vi "FTW-BuildUtil-PostBuildAction.vi"(5 "Files Generated by Build":path[](array[path]), 6 "Top Level/Always Included VIs":path[](array[path]), 7 "Destination Path":path, 8 "error in (no error)":errorcluster, 9 "Target Name":string, 10 "Build Specification Name":string, 11 "Project Path":path) -> (0 "error out":errorcluster)   [LabVIEW 2013]
uses:
  <userlib>/_OpenG.lib/error/error.llb/Filter Error Codes (Array)__ogtk.vi
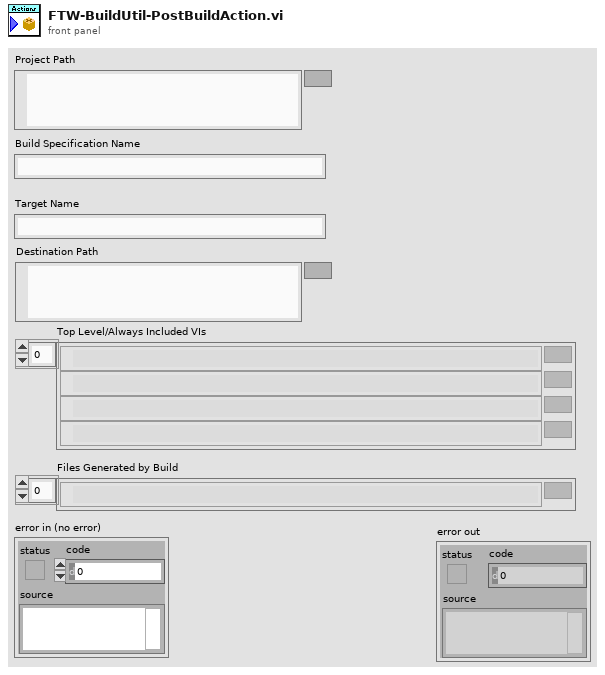
[diagram p1: front panel]
types:
  T1 = cluster{"Major":u16, "Minor":u16, "Fix":u16, "Build":u16}
  T2 = cluster{"Path":path, "lowercase file extension":string, "vi reference":refnum<vi>, "LVClass.Open":refnum<vi>, "Open Library":refnum<vi>}
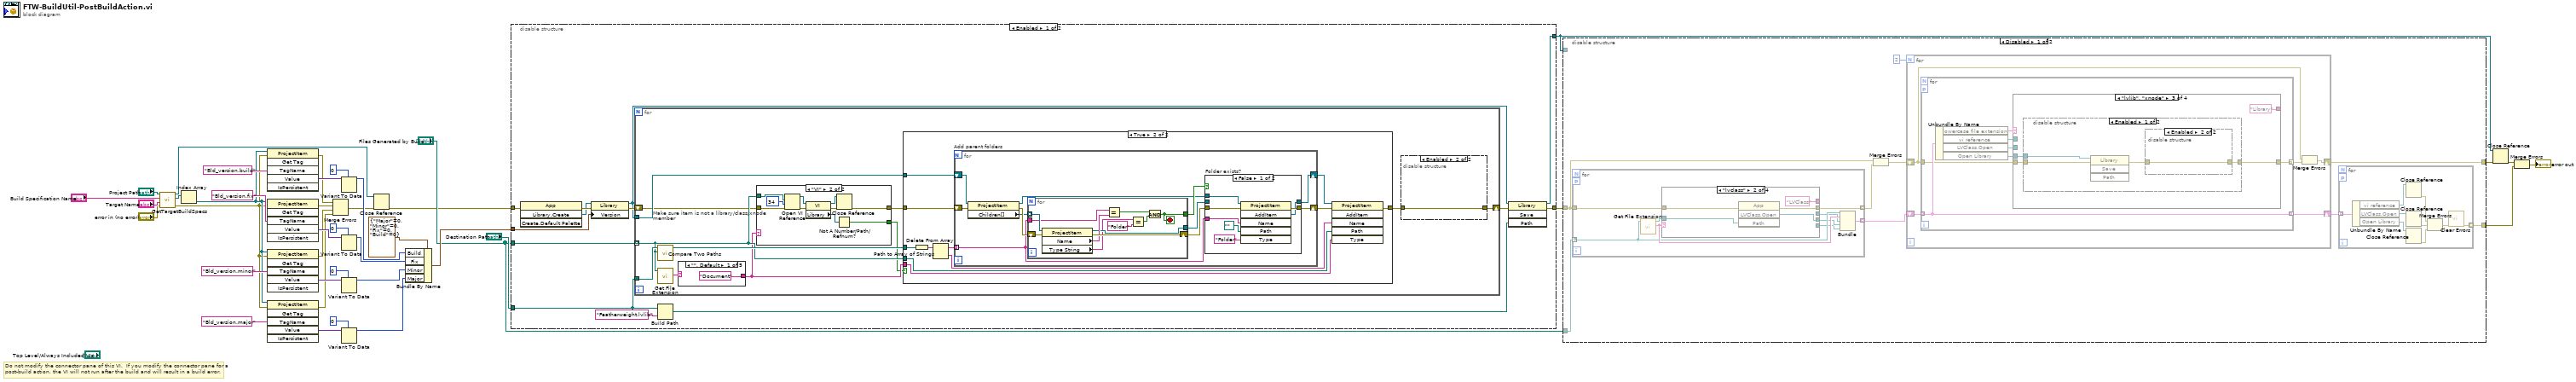
[diagram p0: block diagram]
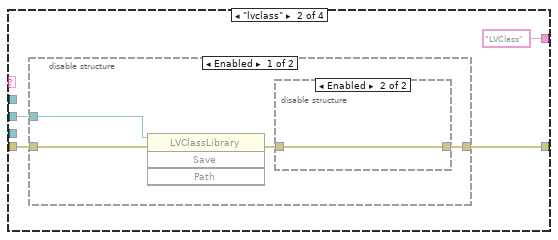
[diagram p3: hidden frame]
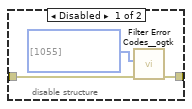
[diagram p4: hidden frame]
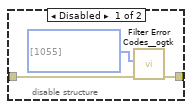
[diagram p6: hidden frame]
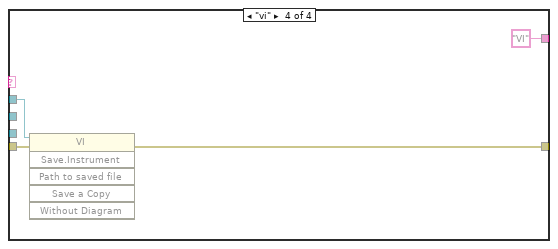
[diagram p8: hidden frame]
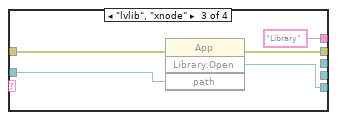
[diagram p10: hidden frame]
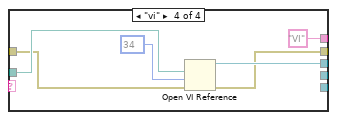
[diagram p11: hidden frame]
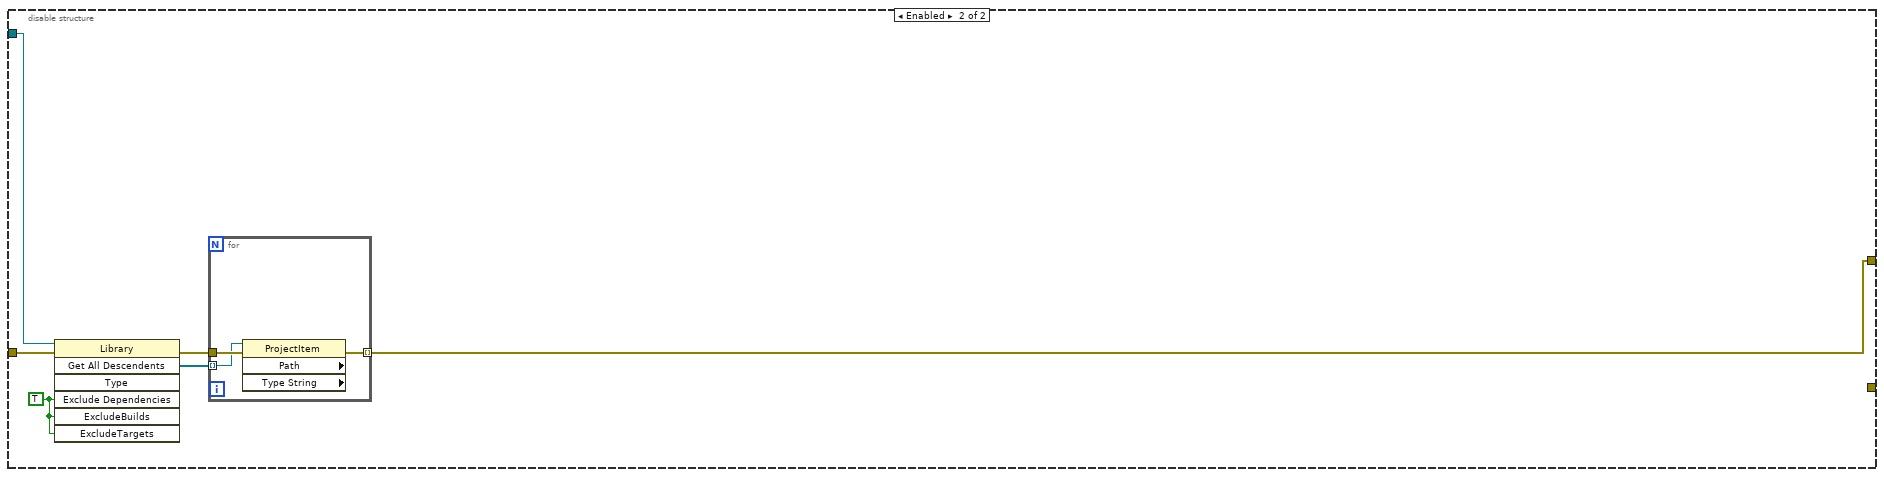
[diagram p12: hidden frame]
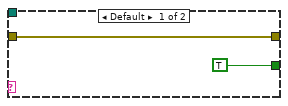
[diagram p15: hidden frame]
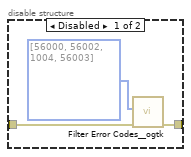
[diagram p16: hidden frame]
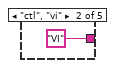
[diagram p17: hidden frame]
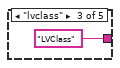
[diagram p18: hidden frame]
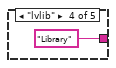
[diagram p19: hidden frame]
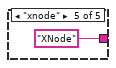
[diagram p20: hidden frame]
diagram:
  # "Do not modify the connector pane of this VI.  If you modify the connector pane for a post-build action, the VI will not run after the build and will result in a build error."
  n1 = call <vilib>:"GetTargetBuildSpecs.vi"("error in (no error)"="error in (no error)", "Name of target (My Computer)"="Target Name", "Name of build specification (if empty: get all)"="Build Specification Name", "Path to project"="Project Path") -> ("error out"=w8:errorcluster, "buildspec refs"=w36:refnum<vi>[], "project ref"=w37:refnum<vi>)  [unwired: 5 in]
  n2 = Index Array(array=w36) -> (element=w9:refnum<vi>)  [unwired: 1 in]
  n3 = invoke class="ProjectItem" method="Get Tag"(reference=w9, error in=w8, "TagName"="Bld_version.build" ("Tag Name")) -> (error out=w22:errorcluster, "Value"=w27:variant)  [unwired: 3 in, 4 out]
  n4 = invoke class="ProjectItem" method="Get Tag"(reference=w9, error in=w8, "TagName"="Bld_version.fix" ("Tag Name")) -> (error out=w7:errorcluster, "Value"=w24:variant)  [unwired: 3 in, 4 out]
  n5 = invoke class="ProjectItem" method="Get Tag"(reference=w9, error in=w8, "TagName"="Bld_version.minor" ("Tag Name")) -> (error out=w6:errorcluster, "Value"=w30:variant)  [unwired: 3 in, 4 out]
  n6 = invoke class="ProjectItem" method="Get Tag"(reference=w9, error in=w8, "TagName"="Bld_version.major" ("Tag Name")) -> (error out=w5:errorcluster, "Value"=w33:variant)  [unwired: 3 in, 4 out]
  n7 = Merge Errors(w22, w7, w6, w5) -> (w10:errorcluster)
  n8 = Variant To Data(type=u16 0, Variant=w27) -> (data=w20:u16)  [unwired: 1 in, 1 out]
  n9 = Variant To Data(type=u16 0, Variant=w24) -> (data=w19:u16)  [unwired: 1 in, 1 out]
  n10 = Variant To Data(type=u16 0, Variant=w30) -> (data=w18:u16)  [unwired: 1 in, 1 out]
  n11 = Variant To Data(type=u16 0, Variant=w33) -> (data=w17:u16)  [unwired: 1 in, 1 out]
  n12 = Close Reference(reference=w37, error in (no error)=w10) -> (error out=w11:errorcluster)
  n13 = Bundle By Name(cluster=T1 {"Major"=0, "Minor"=0, "Fix"=0, "Build"=0} ("Cluster"), "Build"=w20, "Fix"=w19, "Minor"=w18, "Major"=w17) -> (w16:T1)
  n14 = disable-structure shown="Enabled" {
    disable-tunnel: w11 -> [w53 w129]
    disable-tunnel: w16 -> [w50 _]
    disable-tunnel: "Files Generated by Build" -> [w48 _]
    disable-tunnel: "Destination Path" -> [w45 _]
    disable-tunnel: [w42 w129] -> w4
    disable-tunnel: [w41 _] -> w1
    frame Enabled {
      n15 = invoke class="App" method="Library.Create"(error in=w53) -> (error out=w52:errorcluster, "Create Library"=w51:refnum<vi>)  [unwired: 3 in, 2 out]
      n16 = property class="Library"(reference=w51, error in=w52, "Version"=w50) -> (reference out=w46:refnum<vi>, error out=w47:errorcluster)
      n17 = for {
        tunnel: w46 -> [w62]
        shift-right: [w57] -> w49
        shift-left: w47 -> [w56]
        tunnel: w48 -> [w60] mode=indexing
        tunnel: w45 -> [w64]
        n18 = call <vilib>:"Compare Two Paths.vi"("Path 2"=w60, "Path 1"=w64) -> ("Relative Path from 1 to 2"=w63:path)  [unwired: 6 in, 3 out]
        n19 = call <vilib>:"Get File Extension.vi"("file"=w60) -> ("lowercase file extension"=w59:string)  [unwired: 7 in, 3 out]
        n20 = case shown="\"\", Default" w59 {
          tunnel: ["Document" "VI" "LVClass" "Library" "XNode"] -> w58
          frame "", Default {
          }
          frame "ctl", "vi" {
          }
          frame "lvclass" {
          }
          frame "lvlib" {
          }
          frame "xnode" {
          }
        }
        n21 = case "Make sure item is not a library/class/xnode member" shown="\"VI\"" w58 {
          tunnel: [TRUE w114] -> w54
          tunnel: w60 -> [_ w118]
          tunnel: w56 -> [w108 w111]
          tunnel: [w108 w110] -> w55
          frame Default {
          }
          frame "VI" {
            n22 = Open VI Reference(vi path=w118, options=34, error in (no error)=w111) -> (vi reference=w117:refnum<vi>, error out=w116:errorcluster)  [unwired: 3 in]
            n23 = property class="VI"(reference=w117, error in=w116) -> (reference out=w112:refnum<vi>, error out=w113:errorcluster, "Library"=w115:refnum<vi>)
            n24 = Not A Number/Path/Refnum?(number/path/refnum=w115) -> (NaN/Path/Refnum?=w114:bool)
            n25 = Close Reference(reference=w112, error in (no error)=w113) -> (error out=w110:errorcluster)
          }
        }
        n26 = case shown="True" w54 {
          tunnel: w63 -> [_ w76]
          tunnel: w62 -> [_ w75]
          tunnel: [w65 w72] -> w61
          tunnel: w60 -> [_ w69]
          tunnel: w58 -> [_ w68]
          tunnel: w55 -> [w65 w66]
          frame False {
          }
          frame True {
            n27 = Path to Array of Strings(0:w76) -> (2:w73:string[])  [unwired: 1 out]
            n28 = Delete From Array(array=w73) -> (deleted portion=w70:string, array with subset deleted=w74:string[])  [unwired: 2 in]
            n29 = for "Add parent folders" {
              tunnel: w74 -> [w77] mode=indexing
              shift-right: [w80] -> w71
              shift-left: w75 -> [w85]
              shift-right: [w82] -> w67
              shift-left: w66 -> [w87]
              n30 = property class="ProjectItem"(reference=w85, error in=w87) -> (reference out=w78:refnum<vi>, error out=w86:errorcluster, "Children[]"=w83:refnum<vi>[])
              n31 = for {
                tunnel: w83 -> [w105] mode=indexing
                tunnel: w77 -> [w103]
                tunnel: [w98] -> w81
                shift-right: [w106] -> w84
                shift-left: w86 -> [w107]
                tunnel: [w101] -> w79
                stop <- w98 stop-if-true
                n32 = property class="ProjectItem"(reference=w105, error in=w107) -> (reference out=w101:refnum<vi>, error out=w106:errorcluster, "Name"=w104:string, "Type String"=w100:string)
                n33 = Equal?(x=w103, y=w104) -> (x = y?=w102:bool)
                n34 = Equal?(x=w100, y="Folder") -> (x = y?=w97:bool)
                n35 = And(x=w102, y=w97) -> (x .and. y?=w98:bool)
              }
              n36 = case "Folder exists?" shown="False" w81 {
                tunnel: w84 -> [w94 w95]
                tunnel: [w93 w95] -> w82
                tunnel: [w88 w96] -> w80
                tunnel: w79 -> [_ w96]
                tunnel: w78 -> [w92 _]
                tunnel: w77 -> [w90 _]
                frame False {
                  n37 = invoke class="ProjectItem" method="AddItem"(reference=w92, error in=w94, "Name"=w90, "Path"=path "", "Type"="Folder") -> (error out=w93:errorcluster, "AddItem"=w88:refnum<vi>)  [unwired: 1 in, 4 out]
                }
                frame True {
                }
              }
            }
            n38 = invoke class="ProjectItem" method="AddItem"(reference=w71, error in=w67, "Name"=w70, "Path"=w69, "Type"=w68) -> (error out=w72:errorcluster)  [unwired: 1 in, 5 out]
          }
        }
        n39 = disable-structure shown="Enabled" {
          disable-tunnel: w61 -> [w122 w123]
          disable-tunnel: [w121 w123] -> w57
          frame Disabled {
            n40 = call-poly <userlib>:"Filter Error Codes__ogtk.vi"("Error In"=w122, "Error Codes to Filter"=i32[] [56000, 56002, 1004, 56003]) -> ("Error Out"=w121:errorcluster)  [unwired: 7 in, 2 out]
          }
          frame Enabled {
          }
        }
      }
      n41 = Build Path(base path=w45, name or relative path="Featherweight.lvlib") -> (appended path=w43:path)
      n42 = invoke class="Library" method="Save"(reference=w46, error in=w49, "Path"=w43) -> (reference out=w41:refnum<vi>, error out=w42:errorcluster)  [unwired: 1 in, 2 out]
    }
    frame Disabled {
    }
  }
  n43 = disable-structure shown="Disabled" {
    disable-tunnel: "Files Generated by Build" -> [w138 _]
    disable-tunnel: [w133 _] -> w12
    disable-tunnel: w4 -> [w132 w222]
    disable-tunnel: [w134 w218] -> w3
    disable-tunnel: w1 -> [_ w220]
    frame Disabled {
      n44 = for {
        tunnel: w138 -> [w197] mode=indexing
        tunnel: [w195] -> w137 mode=indexing
        tunnel: w132 -> [w194]
        tunnel: [w193] -> w130 mode=indexing
        workers-P: _ -> [_]
        n45 = call <vilib>:"Get File Extension.vi"("file"=w197) -> ("lowercase file extension"=w198:string, "dup file"=w199:path)  [unwired: 7 in, 2 out]
        n46 = case shown="\"lvclass\"" w198 {
          tunnel: [_ "LVClass" "Library" "VI"] -> _
          tunnel: w199 -> [_ w202 w208 w215]
          tunnel: [_ _ _ w213] -> w196
          tunnel: w194 -> [w200 w204 w209 w212]
          tunnel: [w200 w203 w206 w211] -> w193
          tunnel: [_ w201 _ _] -> w192
          tunnel: [_ _ w207 _] -> w191
          frame "", Default {
          }
          frame "lvclass" {
            n47 = invoke class="App" method="LVClass.Open"(error in=w204, "Path"=w202) -> (error out=w203:errorcluster, "LVClass.Open"=w201:refnum<vi>)  [unwired: 2 in, 2 out]
          }
          frame "lvlib", "xnode" {
            n48 = invoke class="App" method="Library.Open"(error in=w209, "path"=w208) -> (error out=w206:errorcluster, "Open Library"=w207:refnum<vi>)  [unwired: 2 in, 2 out]
          }
          frame "vi" {
            n49 = Open VI Reference(vi path=w215, options=34, error in (no error)=w212) -> (vi reference=w213:refnum<vi>, error out=w211:errorcluster)  [unwired: 3 in]
          }
        }
        n50 = Bundle("Path"=w197, "lowercase file extension"=w198, "vi reference"=w196, "LVClass.Open"=w192, "Open Library"=w191) -> (w195:T2)  [unwired: 1 in]
      }
      n51 = Merge Errors(w132, w130) -> (w131:errorcluster)
      n52 = for {
        N: 2 -> [_]
        shift-right: [w141] -> w136
        shift-left: w137 -> [w143]
        shift-right: [w140] -> w134
        shift-left: w131 -> [w139]
        n53 = for {
          tunnel: w143 -> [w150] mode=indexing
          tunnel: [w150] -> w141 mode=indexing
          tunnel: w139 -> [w148]
          tunnel: [w149] -> w142 mode=indexing
          workers-P: _ -> [_]
          n54 = Unbundle By Name(w150) -> ("lowercase file extension"=w146:string, "vi reference"=w147:refnum<vi>, "LVClass.Open"=w145:refnum<vi>, "Open Library"=w144:refnum<vi>)
          n55 = case shown="\"lvlib\", \"xnode\"" w146 {
            tunnel: [_ "LVClass" "Library" "VI"] -> _
            tunnel: w148 -> [w151 w154 w167 w180]
            tunnel: [w151 w152 w165 w179] -> w149
            tunnel: w147 -> [_ _ _ w178]
            tunnel: w145 -> [_ w153 _ _]
            tunnel: w144 -> [_ _ w166 _]
            frame "", Default {
            }
            frame "lvclass" {
              n56 = disable-structure shown="Enabled" {
                disable-tunnel: w154 -> [w159 w164]
                disable-tunnel: w153 -> [w157 _]
                disable-tunnel: [w156 w164] -> w152
                frame Enabled {
                  n57 = invoke class="LVClassLibrary" method="Save"(reference=w157, error in=w159) -> (error out=w158:errorcluster)  [unwired: 2 in, 3 out]
                  n58 = disable-structure shown="Enabled" {
                    disable-tunnel: w158 -> [w162 w163]
                    disable-tunnel: [w161 w163] -> w156
                    frame Disabled {
                      n59 = call-poly <userlib>:"Filter Error Codes__ogtk.vi"("Error In"=w162, "Error Codes to Filter"=i32[] [1055]) -> ("Error Out"=w161:errorcluster)  [unwired: 7 in, 2 out]
                    }
                    frame Enabled {
                    }
                  }
                }
                frame Disabled {
                }
              }
            }
            frame "lvlib", "xnode" {
              n60 = disable-structure shown="Enabled" {
                disable-tunnel: w167 -> [w172 w177]
                disable-tunnel: w166 -> [w171 _]
                disable-tunnel: [w169 w177] -> w165
                frame Enabled {
                  n61 = invoke class="Library" method="Save"(reference=w171, error in=w172) -> (error out=w170:errorcluster)  [unwired: 2 in, 3 out]
                  n62 = disable-structure shown="Enabled" {
                    disable-tunnel: w170 -> [w174 w176]
                    disable-tunnel: [w173 w176] -> w169
                    frame Disabled {
                      n63 = call-poly <userlib>:"Filter Error Codes__ogtk.vi"("Error In"=w174, "Error Codes to Filter"=i32[] [1055]) -> ("Error Out"=w173:errorcluster)  [unwired: 7 in, 2 out]
                    }
                    frame Enabled {
                    }
                  }
                }
                frame Disabled {
                }
              }
            }
            frame "vi" {
              n64 = invoke class="VI" method="Save.Instrument"(reference=w178, error in=w180) -> (error out=w179:errorcluster)  [unwired: 4 in, 5 out]
            }
          }
        }
        n65 = Merge Errors(w139, w142) -> (w140:errorcluster)
      }
      n66 = for {
        tunnel: w136 -> [w190] mode=indexing
        workers-P: _ -> [_]
        tunnel: [w182] -> w133 mode=indexing
        n67 = Unbundle By Name(w190) -> ("vi reference"=w189:refnum<vi>, "LVClass.Open"=w188:refnum<vi>, "Open Library"=w187:refnum<vi>)
        n68 = Close Reference(reference=w189) -> (error out=w186:errorcluster)  [unwired: 1 in]
        n69 = Close Reference(reference=w188) -> (error out=w185:errorcluster)  [unwired: 1 in]
        n70 = Close Reference(reference=w187) -> (error out=w184:errorcluster)  [unwired: 1 in]
        n71 = Merge Errors(w186, w185, w184) -> (w183:errorcluster)
        n72 = call <vilib>:"Clear Errors.vi"("error in (no error)"=w183) -> ("error out"=w182:errorcluster)  [unwired: 6 in]
      }
    }
    frame Enabled {
      w219 = TRUE ("ExcludeDependencies")
      n73 = invoke class="Library" method="Get All Descendents"(reference=w220, error in=w222, "Exclude Dependencies"=w219, "ExcludeBuilds"=w219, "ExcludeTargets"=w219) -> (error out=w221:errorcluster, "All Descendents"=w217:refnum<vi>[])  [unwired: 2 in, 5 out]
      n74 = for {
        tunnel: w221 -> [w225]
        tunnel: [w224] -> w218 mode=indexing
        tunnel: w217 -> [w223] mode=indexing
        n75 = property class="ProjectItem" props=["Path", "Type String"](reference=w223, error in=w225) -> (error out=w224:errorcluster)  [unwired: 3 out]
      }
    }
  }
  n76 = Close Reference(reference=w1, error in (no error)=w3) -> (error out=w2:errorcluster)
  n77 = Merge Errors(w2, w12) -> (→"error out":errorcluster)
